vi "Set ASI LED power.vi"(8 "error in":errorcluster, 10 "New LED power":dbl, 11 "VISA resource in":refnum<visa-resource-name>) -> (0 "error out":errorcluster, 3 "VISA resource name out":refnum<visa-resource-name>)   [LabVIEW 2018]
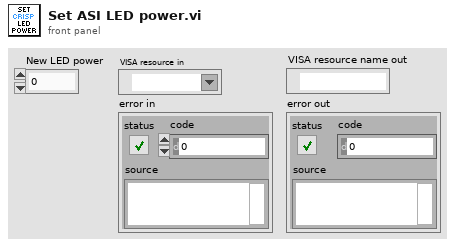
[diagram p1: front panel]
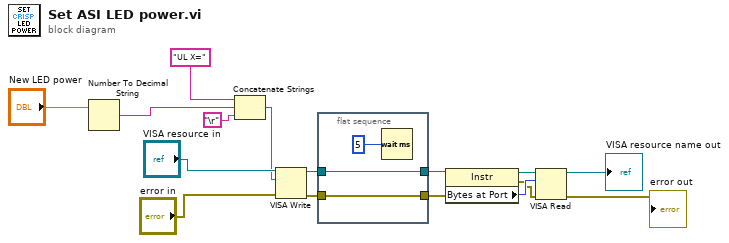
[diagram p0: block diagram]
diagram:
  n1 = Number To Decimal String(number="New LED power") -> (decimal integer string=w1:string)  [unwired: 1 in]
  n2 = Concatenate Strings("UL X=" ("write buffer"), w1, "\r") -> (w6:string)
  n3 = VISA Write(VISA resource name="VISA resource in", write buffer=w6, error in (no error)="error in") -> (VISA resource name out=w13:refnum<visa-resource-name>, error out=w14:errorcluster)  [unwired: 1 out]
  n4 = flat-sequence {
    tunnel: [w19] -> w16
    tunnel: w13 -> [w19]
    tunnel: [w17] -> w15
    tunnel: w14 -> [w17]
    frame #0 {
      n5 = Wait (ms)(milliseconds to wait=u32 5) -> ()  [unwired: 1 out]
    }
  }
  n6 = property class="Instr"(reference=w16, error in=w15) -> (reference out=w12:refnum<visa-resource-name>, error out=w10:errorcluster, "Bytes at Port"=w11:u32)
  n7 = VISA Read(VISA resource name=w12, byte count=w11, error in (no error)=w10) -> (VISA resource name out=→"VISA resource name out":refnum<visa-resource-name>, error out=→"error out":errorcluster)  [unwired: 2 out]
